vi "sendValue.vi"(8 "error in (no error)":errorcluster, 10 "data":variant, 11 "position in":refnum<class "position.lvclass">) -> (0 "error out":errorcluster, 2 "function return":i32, 3 "position out":refnum<class "position.lvclass">)   [LabVIEW 2016, in "SALLV_AtDome_Messaging.lvlib" / "position.lvclass"]
uses:
  position.lvclass
  ts_sallv_AtDome/DataTypes/position.ctl
  ts_sallv_AtDome/SALLV_AtDome.lvlib
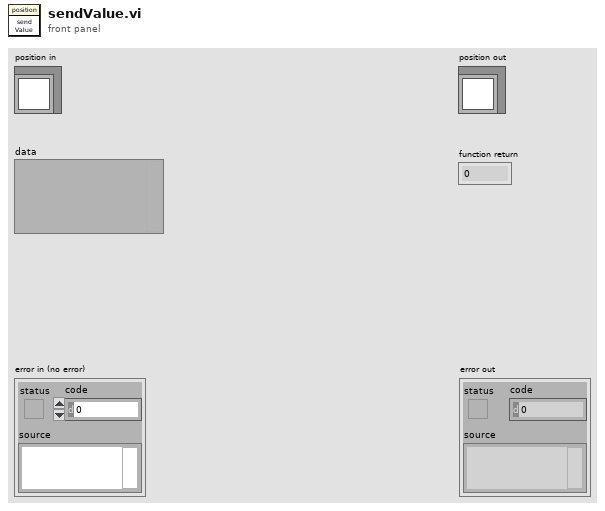
[diagram p1: front panel]
types:
  T1 = typedef "SALLV_AtDome.lvlib/position.ctl" = cluster{"dropoutOpeningPercentage":sgl, "mainDoorOpeningPercentage":sgl, "azimuthPosition":dbl, "dropoutOpeningPercentageSet":sgl, "mainDoorOpeningPercentageSet":sgl, "azimuthPositionSet":dbl}
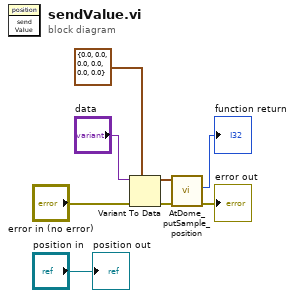
[diagram p0: block diagram]
diagram:
  n1 = Variant To Data(error in="error in (no error)", type=T1 {"dropoutOpeningPercentage"=0.0, "mainDoorOpeningPercentage"=0.0, "azimuthPosition"=0.0, "dropoutOpeningPercentageSet"=0.0, "mainDoorOpeningPercentageSet"=0.0, "azimuthPositionSet"=0.0} ("position_Ctl"), Variant="data") -> (data=w2:T1, error out=w5:errorcluster)
  n2 = call "AtDome_putSample_position.vi"("error in (no error)"=w5, "position_Ctl"=w2) -> ("error out"=→"error out":errorcluster, "function return"=→"function return":i32)  [unwired: 7 in, 1 out]
  "position out" <- "position in"
